vi "LoopScript_SingleVideo.vi"() -> ()   [LabVIEW 2017]
uses:
  FrontPanelReferences.vi
  Desktop/AODExperimentControls/ImageAcquisitionProgram/ImageAcquisitionLibrary/GlobalFrontPanelReferences.vi
  Desktop/AODExperimentControls/ImageAcquisitionProgram/ImageAcquisitionLibrary/ImageAcquisitionLibrary.lvlib
panel:
  out "Current Step Down":i32
  out "Current Step Up":i32
  out "Current Loop":i32
  in  "NumberOfLoops":i32
  in  "Record Time":u32=15000
  in  "B_f^2":dbl
  in  "B_0^2":dbl
  in  "Steps":i32=30
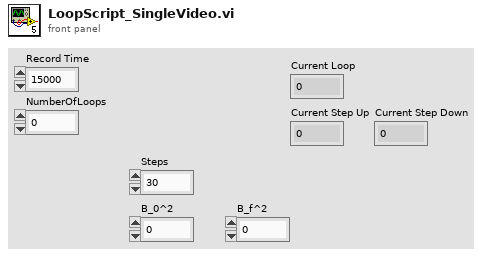
[diagram p1: front panel]
types:
  T1 = typedef "ImageAcquisitionLibrary.lvlib/References.ctl" = cluster{"Acquire":refnum<vi>, "Rec":refnum<vi>, "Tracking":refnum<vi>, "Settings":refnum<vi>, "Stop":refnum<vi>, "Initialized?":bool, "ImDisplay":refnum<vi>}
  T2 = typedef "WaveformGenerator.lvlib/WaveformGeneratorInterfaceRef.ctl" = cluster{"Waveform X":refnum<vi>, "Waveform Y":refnum<vi>, "Waveform Z":refnum<vi>, "Amplitude X":refnum<vi>, "Amplitude Y":refnum<vi>, "Amplitude Z":refnum<vi>, "Frequency X":refnum<vi>, "Frequency Y":refnum<vi>, "Frequency Z":refnum<vi>, "Phase X":refnum<vi>, "Phase Y":refnum<vi>, "Phase Z":refnum<vi>, "Offset X":refnum<vi>, "Offset Y":refnum<vi>, "Offset Z":refnum<vi>, "Stop":refnum<vi>, "On/Off":refnum<vi>, "Field^2":refnum<vi>}
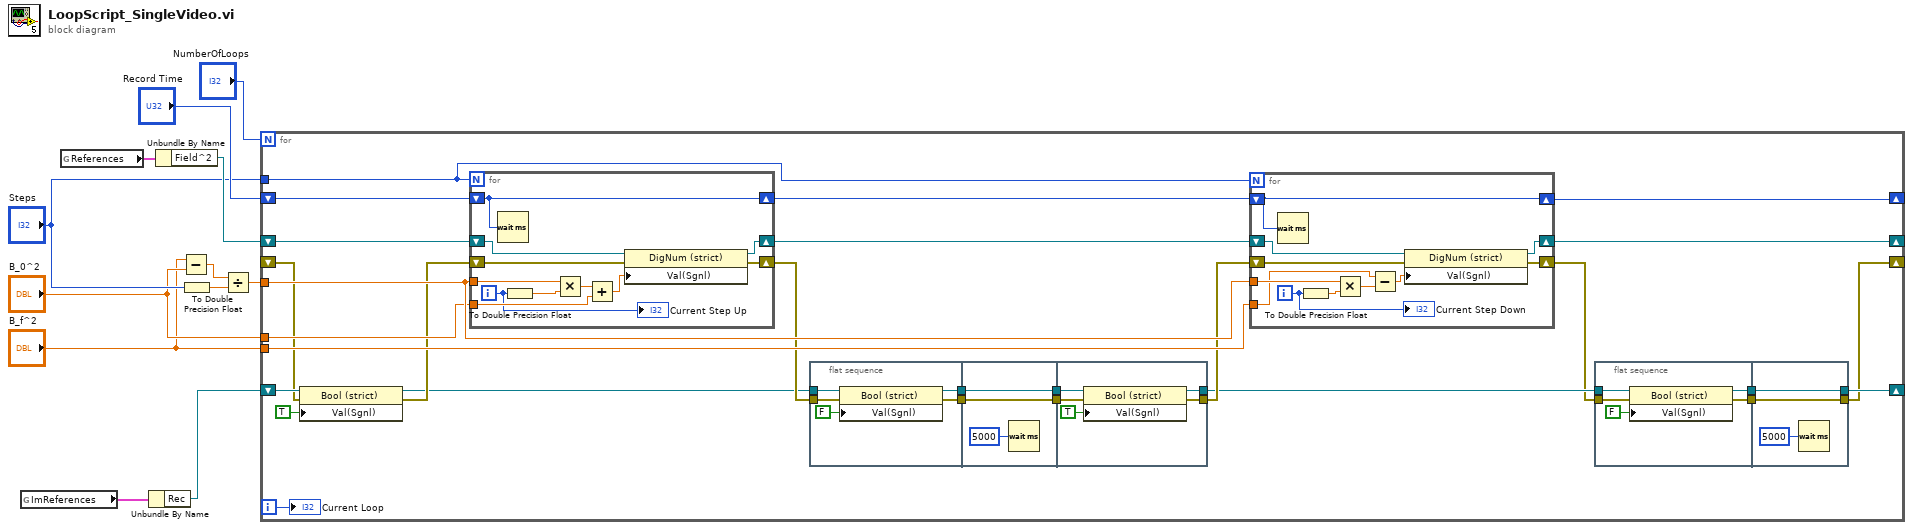
[diagram p0: block diagram]
diagram:
  n1 = global read "GlobalFrontPanelReferences.vi" "ImReferences"() -> (w2:T1)
  n2 = global read "FrontPanelReferences.vi" "References"() -> (w12:T2)
  n3 = Unbundle By Name(w2) -> ("Rec"=w1:refnum<vi>)
  n4 = Unbundle By Name(w12) -> ("Field^2"=w11:refnum<vi>)
  n5 = Subtract(x="B_f^2", y="B_0^2") -> (x-y=w9:dbl)
  n6 = To Double Precision Float(number="Steps") -> (double precision float=w10:dbl)
  n7 = Divide(x=w9, y=w10) -> (x/y=w6:dbl)
  n8 = for {
    N: "NumberOfLoops" -> [_]
    tunnel: "Steps" -> [w38]
    tunnel: w6 -> [w35]
    tunnel: "B_0^2" -> [w34]
    shift-right: [w13] -> _
    shift-left: _ -> [w17]
    shift-right: [w31] -> _
    shift-left: w11 -> [w40]
    shift-right: [w32] -> _
    shift-left: "Record Time" -> [w39]
    tunnel: "B_f^2" -> [w30]
    shift-right: [w15] -> _
    shift-left: w1 -> [w18]
    i -> [w33]
    n9 = property class="Bool (strict)"(reference=w18, error in=w17, "Val(Sgnl)"=TRUE ("Value (Signaling)")) -> (reference out=w20:refnum<vi>, error out=w21:errorcluster)
    n10 = for {
      N: w38 -> [_]
      shift-right: [w76] -> w36
      shift-left: w40 -> [w83]
      shift-right: [w75] -> w29
      shift-left: w21 -> [w82]
      tunnel: w34 -> [w81]
      tunnel: w35 -> [w79]
      shift-right: [w74] -> w37
      shift-left: w39 -> [w74]
      i -> [w73]
      n11 = Wait (ms)(milliseconds to wait=w74) -> ()  [unwired: 1 out]
      n12 = To Double Precision Float(number=w73) -> (double precision float=w80:dbl)
      n13 = Multiply(x=w79, y=w80) -> (x*y=w78:dbl)
      n14 = Add(x=w78, y=w81) -> (x+y=w77:dbl)
      n15 = property class="DigNum (strict)"(reference=w83, error in=w82, "Val(Sgnl)"=w77) -> (reference out=w76:refnum<vi>, error out=w75:errorcluster)
      "Current Step Up" <- w73
    }
    n16 = flat-sequence {
      tunnel: w29 -> [w53]
      tunnel: w20 -> [w52]
      tunnel: [w50] -> w27
      tunnel: [w49] -> w25
      tunnel: [w55] -> w28
      tunnel: w27 -> [w55]
      tunnel: [w54] -> w26
      tunnel: w25 -> [w54]
      tunnel: w28 -> [w61]
      tunnel: w26 -> [w60]
      tunnel: [w58] -> w16
      tunnel: [w57] -> w24
      frame #0 {
        n17 = property class="Bool (strict)"(reference=w52, error in=w53, "Val(Sgnl)"=FALSE ("Value (Signaling)")) -> (reference out=w50:refnum<vi>, error out=w49:errorcluster)
      }
      frame #1 {
        n18 = Wait (ms)(milliseconds to wait=u32 5000) -> ()  [unwired: 1 out]
      }
      frame #2 {
        n19 = property class="Bool (strict)"(reference=w61, error in=w60, "Val(Sgnl)"=TRUE ("Value (Signaling)")) -> (reference out=w58:refnum<vi>, error out=w57:errorcluster)
      }
    }
    n20 = for {
      N: w38 -> [_]
      shift-right: [w68] -> w31
      shift-left: w36 -> [w72]
      shift-right: [w67] -> w14
      shift-left: w24 -> [w71]
      tunnel: w30 -> [w62]
      tunnel: w35 -> [w69]
      shift-right: [w66] -> w32
      shift-left: w37 -> [w66]
      i -> [w64]
      n21 = Wait (ms)(milliseconds to wait=w66) -> ()  [unwired: 1 out]
      n22 = To Double Precision Float(number=w64) -> (double precision float=w70:dbl)
      n23 = Multiply(x=w69, y=w70) -> (x*y=w63:dbl)
      n24 = Subtract(x=w62, y=w63) -> (x-y=w65:dbl)
      n25 = property class="DigNum (strict)"(reference=w72, error in=w71, "Val(Sgnl)"=w65) -> (reference out=w68:refnum<vi>, error out=w67:errorcluster)
      "Current Step Down" <- w64
    }
    n26 = flat-sequence {
      tunnel: w14 -> [w45]
      tunnel: w16 -> [w44]
      tunnel: [w42] -> w23
      tunnel: [w41] -> w22
      tunnel: w23 -> [w47]
      tunnel: w22 -> [w46]
      tunnel: [w47] -> w15
      tunnel: [w46] -> w13
      frame #0 {
        n27 = property class="Bool (strict)"(reference=w44, error in=w45, "Val(Sgnl)"=FALSE ("Value (Signaling)")) -> (reference out=w42:refnum<vi>, error out=w41:errorcluster)
      }
      frame #1 {
        n28 = Wait (ms)(milliseconds to wait=u32 5000) -> ()  [unwired: 1 out]
      }
    }
    "Current Loop" <- w33
  }
